vi "PPR_motor_threshold.vi"(11 "motor in":dbl) -> (3 "motor out":dbl)   [LabVIEW 2019]
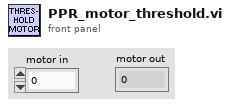
[diagram p1: front panel]
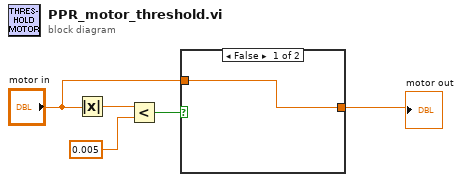
[diagram p0: block diagram]
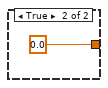
[diagram p2: hidden frame]
diagram:
  n1 = Absolute Value(x="motor in") -> (abs(x)=w5:dbl)
  n2 = Less?(x=w5, y=0.005) -> (x < y?=w3:bool)
  n3 = case shown="False" w3 {
    tunnel: [w6 0.0] -> w2
    tunnel: "motor in" -> [w6 _]
    frame False {
    }
    frame True {
    }
  }
  "motor out" <- w2
